vi "Test_camera_Reconfig.vi"() -> ()   [LabVIEW 2019]
uses:
  <vilib>/vision/driver/IMAQdx.llb/IMAQdx Acquisition Mode.ctl
  <vilib>/vision/driver/NI_Vision_Acquisition_Software.lvlib
panel:
  out "Duration":u32
  in  "Stop":bool
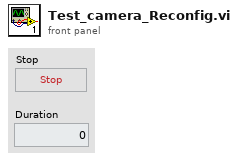
[diagram p1: front panel]
types:
  T1 = typedef "Data.ctl" = cluster{"L16 Linear Actuator":refnum<visa-resource-name>, "XE 1000 Pump":refnum<visa-resource-name>, "Camera1":T2, "Camera2":T2, "Camera1_IMG":T3, "Camera2_IMG":T3, "Img_Capt":bool, "Actuator":bool, "Pump":bool, "Cam 1":bool, "Cam 2":bool, "Empty_Refill":bool, "Crop":bool, "Light intensity":i32, "Exposure Time":dbl, "Sample Name":string, "Operator":string, "Calibration 1":path, "Calibration 2":path, "Framerate":i32, "Timeout Sample":i32, "Collection date":string, "Sample size threshold":i32, "Empty start":u32, "Command":string, "Calibration Image 1":T3, "Calibration Image 2":T3, "Original Image 1":T3, "Original Image 2":T3, "Processing Image 1":T3, "Processing Image 2":T3, "Object Image 1":T3, "Object Image 2":T3, "Station":string, "Species Name":string, "Other Notes":string, "Aperture":enum32{"Item 0", "Item 1", "Item 2", "Item 3"}, "Image Process Queue Size":i32, "Image Save Queue Size":i32, "Overload threshold":i32, "Max Framerate":i32, "Blue Plane Image":T3, "Subtract Image":T3, "Binary Image 1":T3, "ROI mask allocation":T3, "Rectangle 1":T4, "Rectangle 2":T4, "Binary Image 2":T3, "Detection Region %":dbl, "Cam 1 queue":refnum<queue>, "Cam 2 queue":refnum<queue>, "Detect image 1":T3, "Detect image 2":T3, "Detect 1":path, "Detect 2":path, "Max large object threshold":i32, "Open(T)/Close(F)":bool, "Cam 1 - save queue":refnum<queue>, "Cam 2 - save queue":refnum<queue>, "Img_Capt Begin":bool}
  T2 = typedef "IMAQdx.ctl" = refnum<k21>
  T3 = typedef "IMAQ Image.ctl" = refnum<image>
  T4 = typedef "IMAQ Rectangle" = cluster{"Left":i32, "Top":i32, "Right":i32, "Bottom":i32, "Rotation":dbl}
  T5 = typedef "NI_Vision_Acquisition_Software.lvlib/IMAQdx Acquisition Mode.ctl" = enum32{"One Shot", "Continuous"}
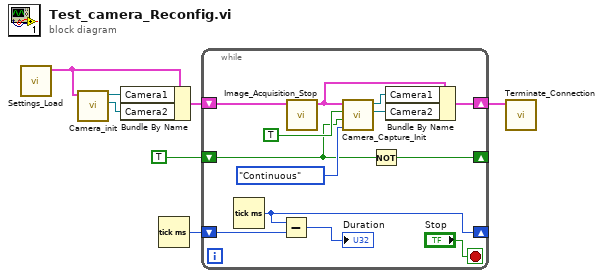
[diagram p0: block diagram]
diagram:
  n1 = call "Settings_Load.vi"() -> ("value"=w1:T1)  [unwired: 10 in, 1 out]
  n2 = call "Camera_init.vi"("input cluster"=w1) -> ("Camera2"=w6:T2, "Camera1"=w7:T2)  [unwired: 7 in, 2 out]
  n3 = Bundle By Name(cluster=w1, "Camera1"=w7, "Camera2"=w6) -> (w5:T1)
  n4 = Tick Count (ms)() -> (millisecond timer value=w3:u32)
  n5 = while {
    shift-right: [w14] -> w4
    shift-left: w5 -> [w15]
    shift-right: [w12] -> _
    shift-left: w3 -> [w11]
    shift-right: [w9] -> _
    shift-left: TRUE -> [w8]
    stop <- "Stop" stop-if-true
    n6 = Tick Count (ms)() -> (millisecond timer value=w12:u32)
    n7 = Subtract(x=w12, y=w11) -> (x-y=→"Duration":u32)
    n8 = call "Image_Acquisition_Stop.vi"("input cluster"=w15) -> ("output cluster"=w16:T1)  [unwired: 10 in]
    n9 = call "Camera_Capture_Init.vi"("Continuous?"=IMAQdx_Acquisition_Mode."Continuous", "Detect Movement"=w8, "Crop?"=TRUE, "input cluster"=w16) -> ("Camera2"=w17:T2, "Camera1"=w18:T2)  [unwired: 6 in]
    n10 = Not(x=w8) -> (.not. x?=w9:bool)
    n11 = Bundle By Name(cluster=w16, "Camera1"=w18, "Camera2"=w17) -> (w14:T1)
  }
  n12 = call "Terminate_Connection.vi"("Data"=w4) -> ()  [unwired: 9 in, 2 out]
